vi "permutation.vi"(11 "P":i32[][](array[numeric])) -> (3 "permutation":i32[](array[numeric]))   [LabVIEW 2014]
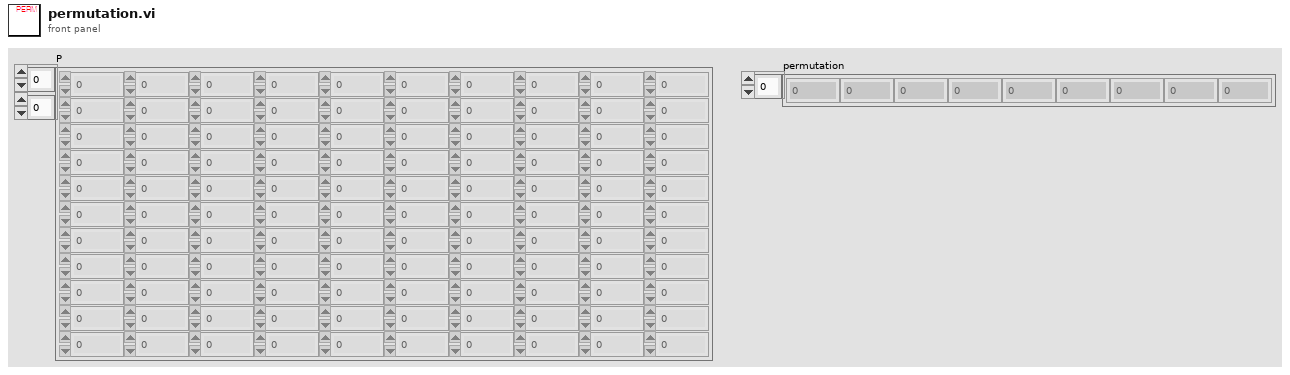
[diagram p1: front panel]
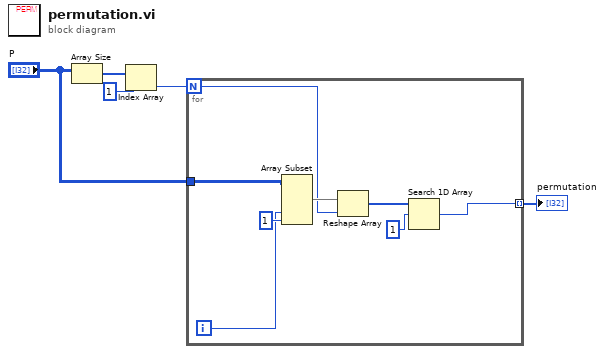
[diagram p0: block diagram]
diagram:
  n1 = Array Size(array="P") -> (size(s)=w5:i32[])
  n2 = Index Array(array=w5, index=1) -> (element=w3:i32)
  n3 = for {
    N: w3 -> [w11]
    tunnel: "P" -> [w13]
    tunnel: [w6] -> w1 mode=indexing
    i -> [w9]
    n4 = Array Subset(array=w13, index (col)=w9, length (col)=1 ("length")) -> (w12:i32[][])  [unwired: 2 in]
    n5 = Reshape Array(w12, w11) -> (w7:i32[])
    n6 = Search 1D Array(1D array=w7, element=1) -> (index of element=w6:i32)  [unwired: 1 in]
  }
  "permutation" <- w1
